vi "Test Constructor.vi"(8 "error in":errorcluster, 11 "data in":T1) -> (0 "error out":errorcluster, 2 "data out":T1, 3 "session reservation out":refnum<class "Session Reservation.lvclass">)   [LabVIEW 2020, in "MeasurementLink Session Management V1.lvlib" / "Session Reservation.lvclass"]
uses:
  Session Reservation.lvclass
  Data.ctl
  Connection Map/Connection Map.lvclass
  IReservation Observer/IReservation Observer.lvclass
  Session and Driver Info.ctl
  MeasurementLink Instrument/ISession Factory/ISession Factory.lvclass
  Generated/Measurement Plugin Session Management Client/RPC Messages/ni_measurementlink_sessionmanagement_v1_SessionInformation.ctl
  Generated/Measurement Plugin Session Management Client/RPC Messages/nidevice_grpc_Session.ctl
  Generated/Measurement Plugin Session Management Client/RPC Messages/ni_measurementlink_sessionmanagement_v1_ChannelMapping.ctl
  MeasurementLink Instrument/ISession Factory/Initialize and Close Session Behavior.ctl
  Generated/Measurement Plugin Session Management Client/RPC Messages/ni_measurementlink_PinMapContext.ctl
  Group Mapping.ctl
  Session Reservation.lvclass/Session Reservation.ctl
  Generated/Measurement Plugin Session Management Client/MeasurementLink Session Management Client.lvlib
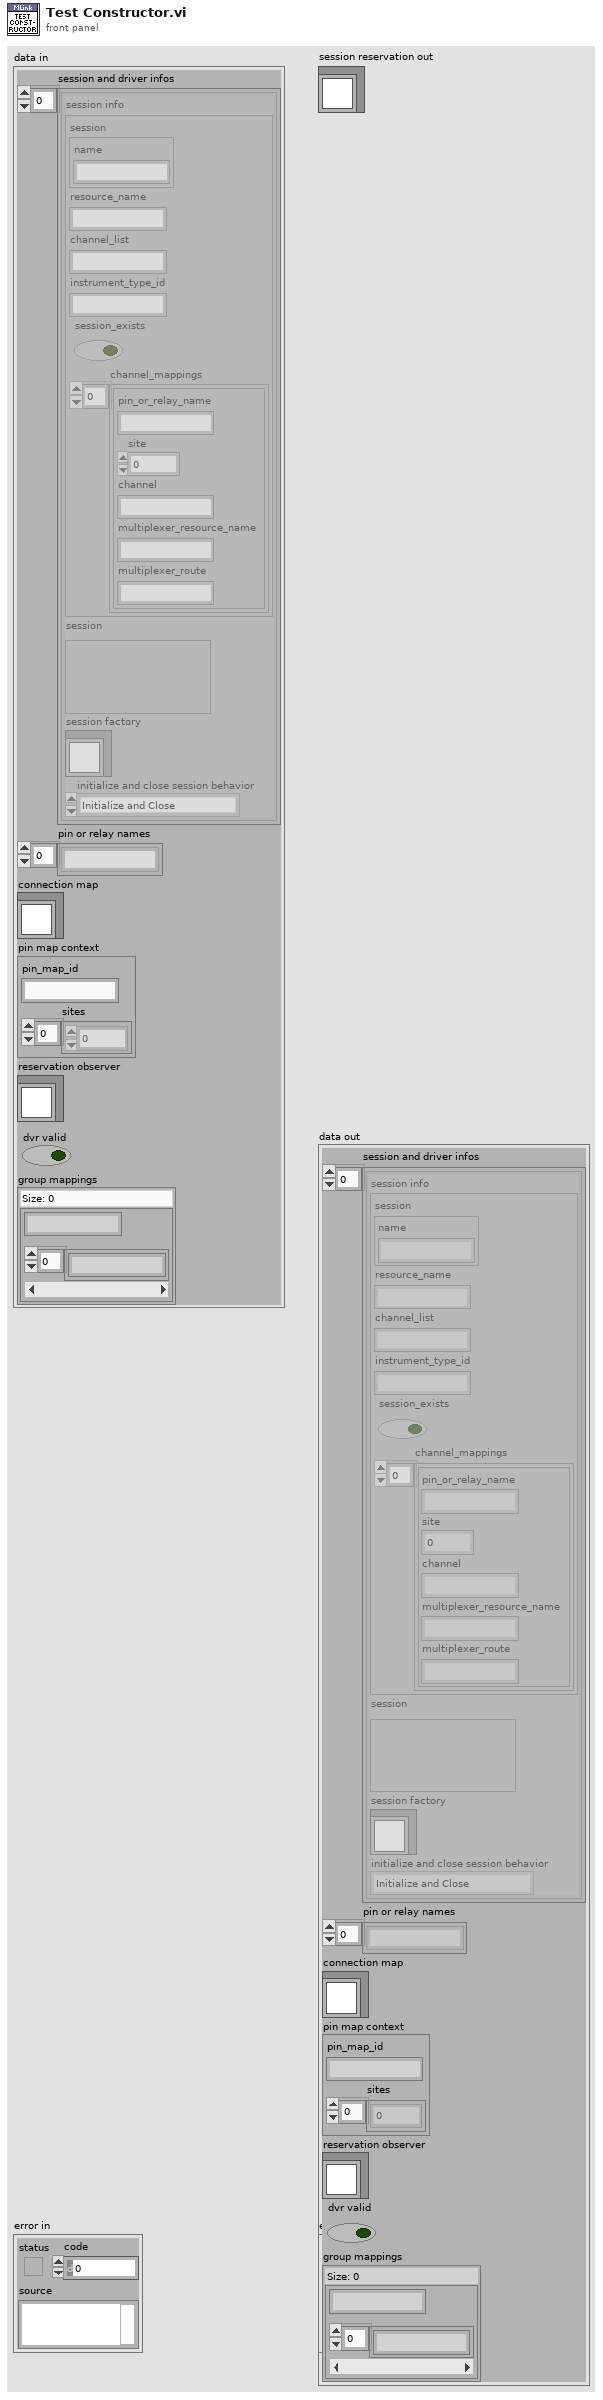
[diagram p1: front panel]
types:
  T1 = typedef "MeasurementLink Session Management V1.lvlib/Session Reservation.lvclass/Data.ctl" = cluster{"session and driver infos":T2[], "pin or relay names":string[], "connection map":refnum<class "Connection Map.lvclass">, "pin map context":T7, "reservation observer":refnum<class "IReservation Observer.lvclass">, "dvr valid":bool, "group mappings":T8}
  T2 = typedef "MeasurementLink Session Management V1.lvlib/Session Reservation.lvclass/Session and Driver Info.ctl" = cluster{"session info":T3, "session":variant, "session factory":refnum<class "ISession Factory.lvclass">, "initialize and close session behavior":T6}
  T3 = typedef "MeasurementLink Session Management Client.lvlib/ni_measurementlink_sessionmanagement_v1_SessionInformation.ctl" = cluster{"session":T4, "resource_name":string, "channel_list":string, "instrument_type_id":string, "session_exists":bool, "channel_mappings":T5[]}
  T4 = typedef "MeasurementLink Session Management Client.lvlib/nidevice_grpc_Session.ctl" = cluster{"name":string}
  T5 = typedef "MeasurementLink Session Management Client.lvlib/ni_measurementlink_sessionmanagement_v1_ChannelMapping.ctl" = cluster{"pin_or_relay_name":string, "site":i32, "channel":string, "multiplexer_resource_name":string, "multiplexer_route":string}
  T6 = typedef "MeasurementLink Instrument.lvlib/ISession Factory.lvclass/Initialize and Close Session Behavior.ctl" = enum16{"Initialize and Close", "Attach and Detach", "Initialize and Detach", "Attach and Close"}
  T7 = typedef "MeasurementLink Session Management Client.lvlib/ni_measurementlink_PinMapContext.ctl" = cluster{"pin_map_id":string, "sites":i32[]}
  T8 = typedef "MeasurementLink Session Management V1.lvlib/Session Reservation.lvclass/Group Mapping.ctl" = map{string, string[]}
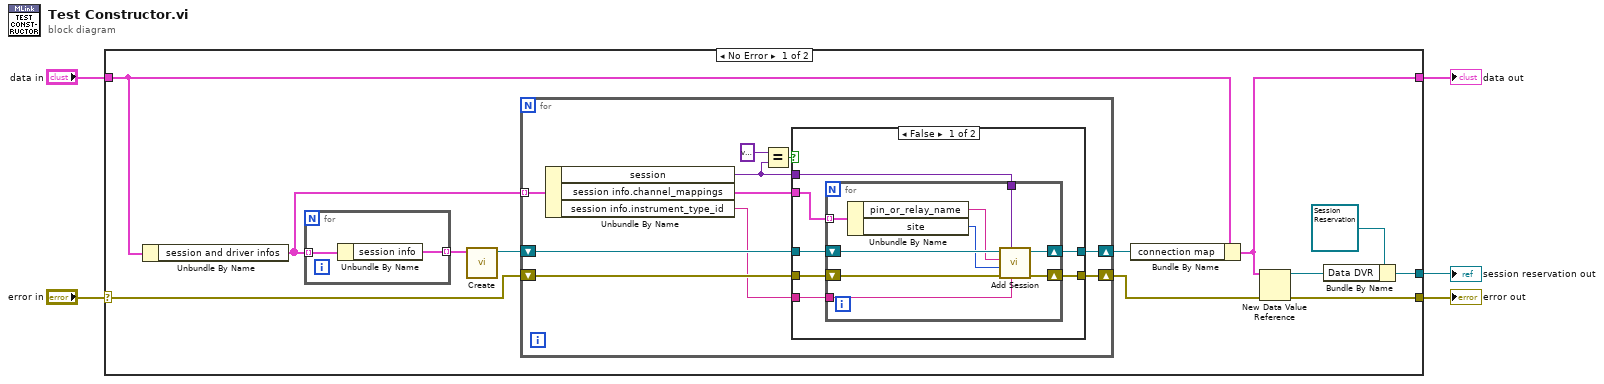
[diagram p0: block diagram]
diagram:
  n1 = case shown="No Error" "error in" {
    selector: "error in" -> [w9 w49]
    tunnel: [w15 w49] -> w4
    tunnel: "data in" -> [w12 w48]
    tunnel: [w14 _] -> w2
    tunnel: [w6 w48] -> w1
    frame No Error {
      n2 = Unbundle By Name(w12) -> ("session and driver infos"=w11:T2[])
      n3 = for {
        tunnel: w11 -> [w47] mode=indexing
        tunnel: [w46] -> w13 mode=indexing
        n4 = Unbundle By Name(w47) -> ("session info"=w46:T3)
      }
      n5 = call "Create.vi"("session info"=w13) -> ("connection map"=w10:refnum<class "Connection Map.lvclass">)  [unwired: 10 in]
      n6 = for {
        tunnel: w11 -> [w27] mode=indexing
        shift-right: [w23] -> w7
        shift-left: w10 -> [w25]
        shift-right: [w21] -> w8
        shift-left: w9 -> [w22]
        n7 = Unbundle By Name(w27) -> ("session"=w20:variant, "session info.channel_mappings"=w19:T5[], "session info.instrument_type_id"=w18:string)
        n8 = Equal?(x=variant ("session"), y=w20) -> (x = y?=w24:bool)
        n9 = case shown="False" w24 {
          tunnel: w25 -> [w34 w45]
          tunnel: [w33 w45] -> w23
          tunnel: w22 -> [w32 w44]
          tunnel: [w31 w44] -> w21
          tunnel: w20 -> [w30 _]
          tunnel: w19 -> [w28 _]
          tunnel: w18 -> [w29 _]
          frame False {
            n10 = for {
              tunnel: w30 -> [w39]
              tunnel: w29 -> [w38]
              shift-right: [w42] -> w33
              shift-left: w34 -> [w43]
              shift-right: [w40] -> w31
              shift-left: w32 -> [w41]
              tunnel: w28 -> [w37] mode=indexing
              n11 = Unbundle By Name(w37) -> ("pin_or_relay_name"=w36:string, "site"=w35:i32)
              n12 = call "Add Session.vi"("instrument type id"=w38, "session to add"=w39, "error in"=w41, "site"=w35, "pin or relay name"=w36, "connection map in"=w43) -> ("error out"=w40:errorcluster, "connection map out"=w42:refnum<class "Connection Map.lvclass">)  [unwired: 4 in]
            }
          }
          frame True {
          }
        }
      }
      n13 = Bundle By Name(cluster=w12, "connection map"=w7) -> (w6:T1)
      n14 = New Data Value Reference(data value=w6, error in=w8) -> (data value reference=w16:refnum<data-value>, error out=w15:errorcluster)
      n15 = Bundle By Name(cluster=refnum<class "Session Reservation.lvclass"> refnum ("MeasurementLink Session Management.lvlib:Session Reservation.lvclass"), "Data DVR"=w16) -> (w14:refnum<class "Session Reservation.lvclass">)
    }
    frame Error {
    }
  }
  "error out" <- w4
  "session reservation out" <- w2
  "data out" <- w1
